vi "BOM Length.vi"(8 "error in (no error)":errorcluster, 11 "String in":string) -> (0 "error out":errorcluster, 3 "String out":string)   [LabVIEW 2019, in "JKI Unicode.lvlib" / "UTF-8 String.lvclass"]
doc: "JKI Unicode 1.0.0.7\nTomi Maila - JKI\nCopyright (c) 2016, JKI"
uses:
  UTF-8 String.lvclass
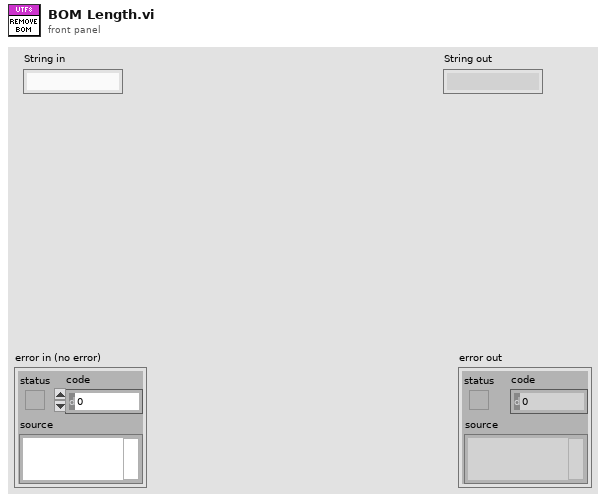
[diagram p1: front panel]
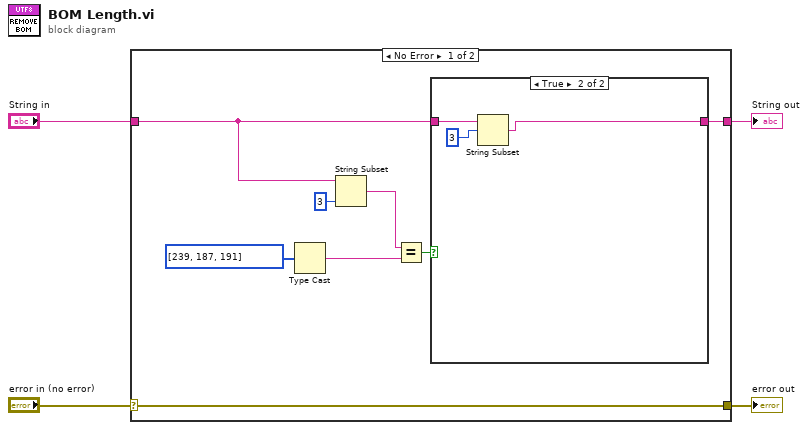
[diagram p0: block diagram]
diagram:
  n1 = case shown="No Error" "error in (no error)" {
    selector: "error in (no error)" -> [w12 w18]
    tunnel: [w12 w18] -> w3
    tunnel: "String in" -> [w6 w17]
    tunnel: [w5 w17] -> w1
    frame No Error {
      n2 = Type Cast(x=u8[] [239, 187, 191]) -> (*(type *) &x=w9:string)  [unwired: 1 in]
      n3 = String Subset(string=w6, length (rest)=3 ("length (rest)")) -> (substring=w8:string)  [unwired: 1 in]
      n4 = Equal?(x=w8, y=w9) -> (x = y?=w7:bool)
      n5 = case shown="True" w7 {
        tunnel: w6 -> [w13 w16]
        tunnel: [w13 w15] -> w5
        frame False {
        }
        frame True {
          n6 = String Subset(string=w16, offset (0)=3) -> (substring=w15:string)  [unwired: 1 in]
        }
      }
    }
    frame Error {
    }
  }
  "error out" <- w3
  "String out" <- w1
